vi "PKG_IMC_InstallEvent.vi"(0 "Handle":u32, 1 "Src1_axis":i16, 2 "Src2_axis":i16, 3 "dest_loc":i16, 5 "EventCMD":i16, 7 "EventType":i16, 8 "EventNum":i32, 9 "Src1_loc":i16, 10 "reserve":i32, 12 "Src2_loc":i16, 13 "reserve":i32, 14 "dest_axis":i16) -> (4 "Handle out":u32, 6 "function return":i32)   [LabVIEW 2011, in "IMC_Pkg4xxx.lvlib"]
doc: "PKG_IMC_InstallEvent(IMC_HANDLE Handle, EventInfo pEvent[], int EventNum );"
uses:
  IMC_Pkg4xxx.lvlib
  IMC_Pkg4xxx.dll
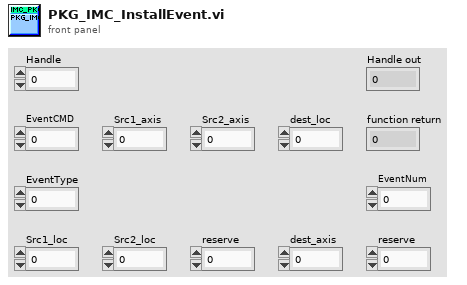
[diagram p1: front panel]
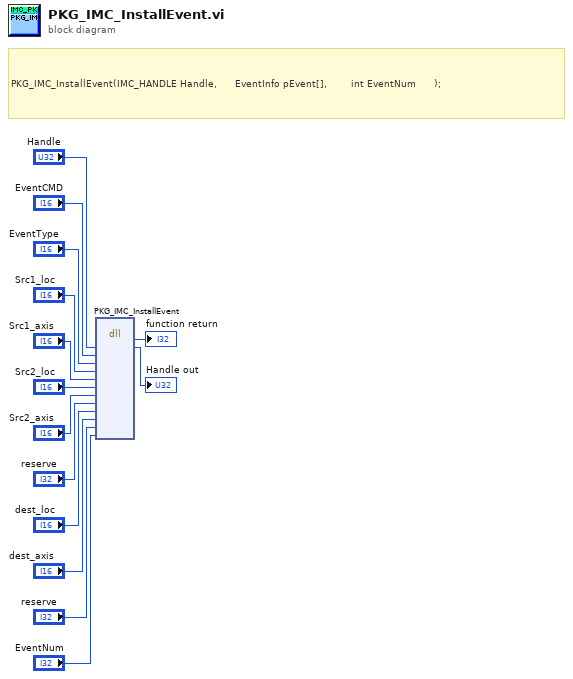
[diagram p0: block diagram]
diagram:
  # "PKG_IMC_InstallEvent(IMC_HANDLE Handle, \t\t\t\t\tEventInfo pEvent[], \t\t\t\t\t\t\tint EventNum\t\t\t\t\t\t);"
  n1 = dll-call lib="PTH1mabs F光盘刻录\niMC MotionIMCNet_V4.0IMCAppincLabviewIMC_PKG4xxxIMC_PKG4xxx\nIMC_Pkg4xxx.*" fn="PKG_IMC_InstallEvent"("Handle"="Handle", "EventCMD"="EventCMD", "EventType"="EventType", "Src1_loc"="Src1_loc", "Src1_axis"="Src1_axis", "Src2_loc"="Src2_loc", "Src2_axis"="Src2_axis", "reserve"="reserve", "dest_loc"="dest_loc", "dest_axis"="dest_axis", "reserve"="reserve", "EventNum"="EventNum") -> (→"function return":i32, "Handle"=→"Handle out":u32)  [unwired: 14 in, 2 out]
